vi "Pixels Per Micron For All FoV.vi"() -> ()   [LabVIEW 2020]
uses:
  <vilib>/vision/Measure.llb/Edge Options.ctl
  <vilib>/vision/Measure.llb/Edge Polarity.ctl
  <vilib>/Analysis/baseanly.llb/Mean (DBL).vi
  <vilib>/Utility/file.llb/Write Delimited Spreadsheet (DBL).vi
  <vilib>/vision/NI_Vision_Development_Module.lvlib
  <vilib>/Analysis/NI_AALBase.lvlib
panel:
  in  "Threshold Data":T1(array[cluster])=[{"Lower value"=140.0, "Upper value"=255.0, "Replace Value"=0.0, "Keep/Replace Value (Replace)"=FALSE}, {"Lower value"=140.0, "Upper value"=255.0, "Replace Value"=255.0, "Keep/Replace Value (Replace)"=TRUE}] {"Replace Value" format="%.2f"; "Upper value" format="%.2f"; "Lower value" format="%.2f"}
  out "output cluster":cluster{i32[], dbl[]}(graph)={[5, 6, 7, 8, 9, 10, 11, 12, 13, 14, 15, 16, 17, 18, 19, 20, 21, 22, 23, 24, 25, 26, 27, 28, 29, 30, 31, 32, 33, 34, 35, 36, 37, 38, 39, 40, 41, 42, 43, 44, 45, 46, 47, 48, 49, 50, 51, 52, 53, 54, 55, 56, 57, 58, 59, 60, 61, 62, 63, 64, 65, 66, 67, 68, 69, 70, 71, 72, 73, 74, 75, 76, 77, 78], [6.014901123046875, 0.0, 26.758624267578124, 14.584745788574219, 23.696197509765625, 0.0, 5.14136962890625, 33.5981689453125, 13.677774047851562, 24.873800659179686, 0.0, 30.73720703125, nan, 0.0, 35.932763671875, 0.0, nan, nan, 18.756075032552083, 0.0, 5.87806282043457, nan, 35.273126220703126, 2.967665100097656, 2.766326904296875, 9.08037872314453, nan, nan, nan, 38.17447204589844, nan, 0.0, 0.0, 12.061470031738281, nan, nan, nan, nan, nan, 0.0, nan, 23.260025024414062, nan, nan, nan, nan, 0.0, nan, 0.0, 0.0, 18.1035888671875, nan, nan, nan, 30.044448852539062, 8.698919677734375, nan, 0.0, nan, nan, nan, 47.926483154296875, nan, nan, nan, nan, nan, nan, nan, nan, nan, 17.186370849609375, nan, nan]}
  in  "Size & Tolerance":T2={"X Size"=5, "Y Size"=5, "% Tolerance"=10}
  in  "ROI":T3={"Global Rectangle"=[0, 0, 1023, 1023], "Contours"=[{"ID"=enum."External", "Type"=3, "Coordinates"=[0, 100, 1023, 900]}]} {"Contours"."Type" items=["No Selection", "Point", "Line", "Rectangle", "Oval", "Polygon", "Freehand Region", "Annulus", "Unused2", "Unused3", "Broken Line", "Freehand Line", "Rotated Rectangle"]}
  in  "Options":T6={"Search Direction"=0, "Edge Options"={"Edge Polarity"=1, "Kernel Size"=3, "Width"=7, "Minimum Edge Strength"=50.0, "Interpolation Type"=enum."Bilinear Fixed", "Data Processing Method"=enum."Average"}, "Show Search Area"=FALSE, "Show Search Lines"=FALSE, "Show Edges Found"=FALSE, "Show Result"=TRUE, "Search Area Color"=65280, "Search Lines Color"=255, "Edge Locations Color"=16776960, "Result Color"=16711680, "Overlay Group Name"=""} {"Search Direction" items=["Left to Right", "Right to Left", "Top to Bottom", "Bottom to Top"]; "Edge Options"."Edge Polarity" items=["All Edges", "Rising Edges", "Falling Edges"]; "Edge Options"."Minimum Edge Strength" format="%.2f"; "Edge Options"."Width" step=2; "Edge Options"."Kernel Size" step=2}
  out "Image":T7(plugin-control)
  in  "File Path":path=path "D:/Data/Calibration/2023/Zoom Cal 10um with correct Align/TIFFs"
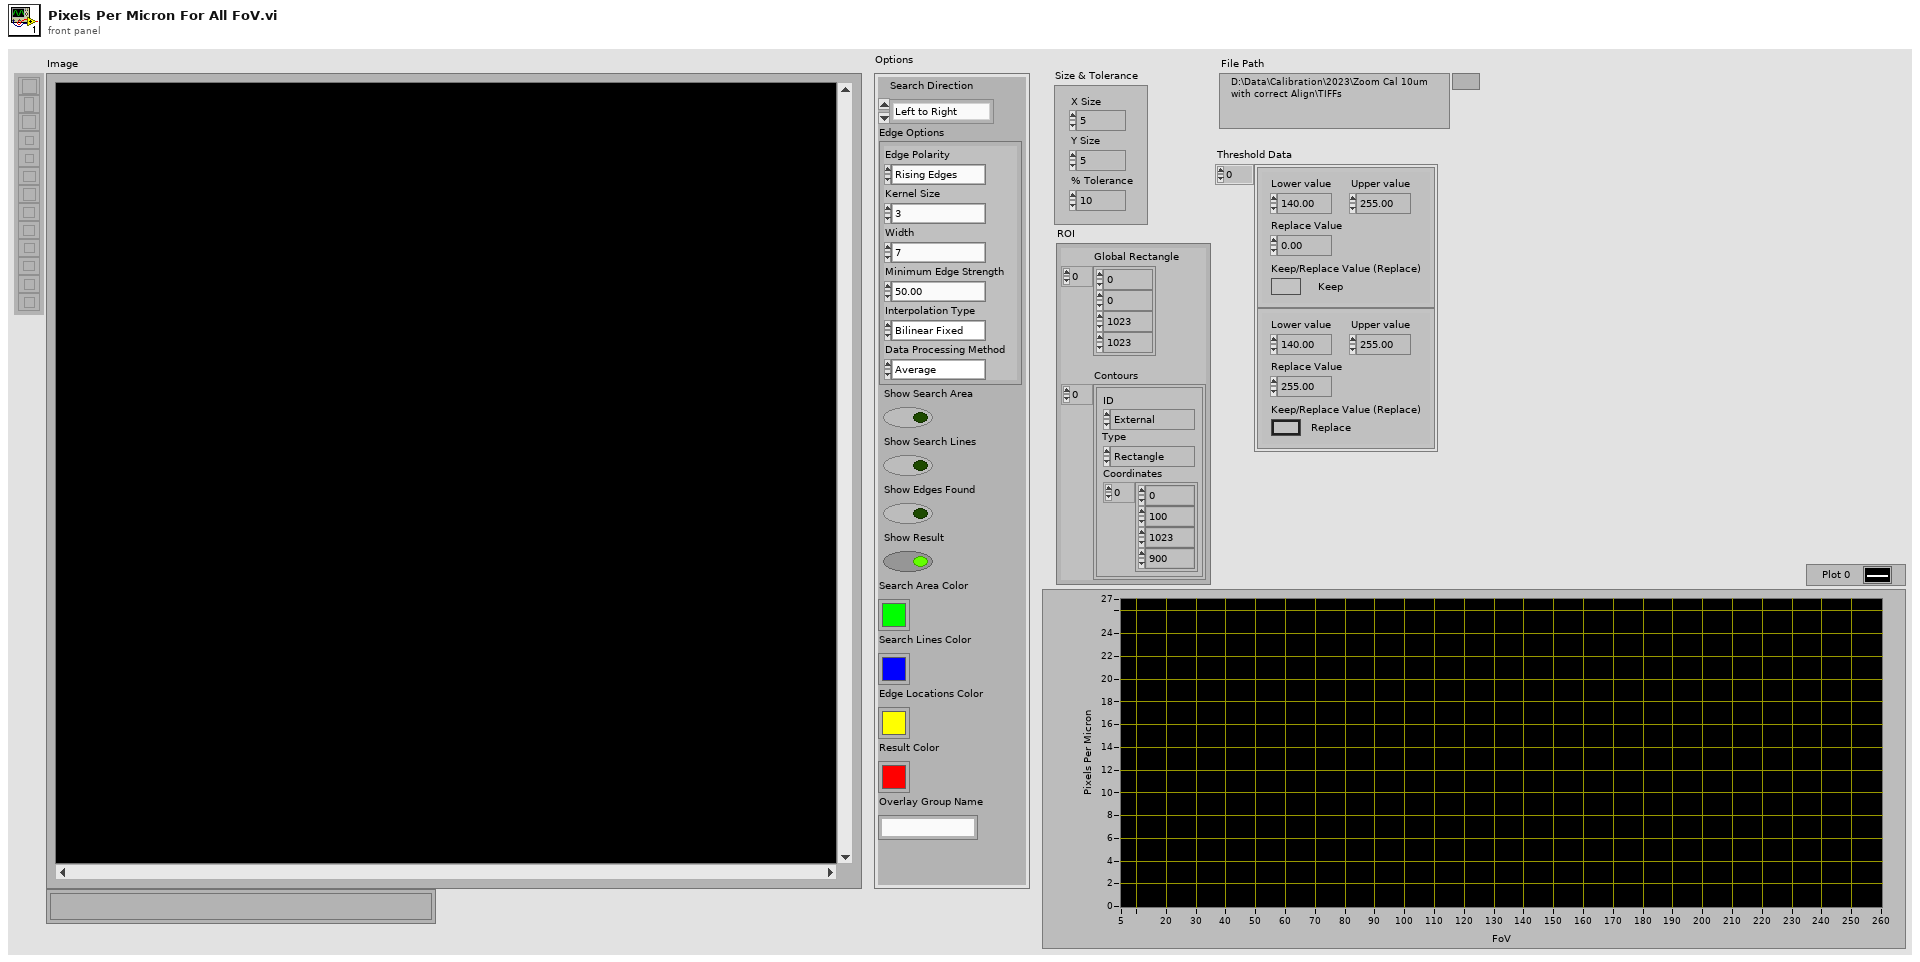
[diagram p1: front panel]
types:
  T1 = cluster{"Lower value":sgl, "Upper value":sgl, "Replace Value":sgl, "Keep/Replace Value (Replace)":bool}[]
  T2 = cluster{"X Size":i32, "Y Size":i32, "% Tolerance":i32}
  T3 = typedef "ROI Descriptor" = cluster{"Global Rectangle":i32[], "Contours":cluster{"ID":enum32{"External", "Internal"}, "Type":u32, "Coordinates":i32[]}[]}
  T4 = typedef "Edge Options.ctl" = cluster{"Edge Polarity":T5, "Kernel Size":u32, "Width":u32, "Minimum Edge Strength":sgl, "Interpolation Type":enum32{"Zero Order", "Bilinear", "Quadratic", "Cubic", "Bilinear Fixed"}, "Data Processing Method":enum32{"Average", "Median"}}
  T5 = typedef "Edge Polarity.ctl" = u32
  T6 = cluster{"Search Direction":u32, "Edge Options":T4, "Show Search Area":bool, "Show Search Lines":bool, "Show Edges Found":bool, "Show Result":bool, "Search Area Color":u32, "Search Lines Color":u32, "Edge Locations Color":u32, "Result Color":u32, "Overlay Group Name":string}
  T7 = typedef "IMAQ Image.ctl" = refnum<image>
  T8 = typedef "Image Type" = u32
  T9 = cluster{"ID":enum32{"External", "Internal"}, "Type":u32, "Coordinates":i32[]}[]
  T10 = cluster{"ID":enum32{"External", "Internal"}, "Type":u32, "Coordinates":i32[]}
  T11 = cluster{"Point1 (Pixels)":cluster{"X":sgl, "Y":sgl}, "Point2 (Pixels)":cluster{"X":sgl, "Y":sgl}, "Point1 (Real-World)":cluster{"X":sgl, "Y":sgl}, "Point2 (Real-World)":cluster{"X":sgl, "Y":sgl}, "Angle (Pixel)":dbl, "Angle (Real-World)":dbl, "Score":dbl, "Straightness":dbl, "Average SNR (db)":dbl, "Calibration Valid":bool}[]
  T12 = cluster{"Point1 (Pixels)":cluster{"X":sgl, "Y":sgl}, "Point2 (Pixels)":cluster{"X":sgl, "Y":sgl}, "Point1 (Real-World)":cluster{"X":sgl, "Y":sgl}, "Point2 (Real-World)":cluster{"X":sgl, "Y":sgl}, "Angle (Pixel)":dbl, "Angle (Real-World)":dbl, "Score":dbl, "Straightness":dbl, "Average SNR (db)":dbl, "Calibration Valid":bool}
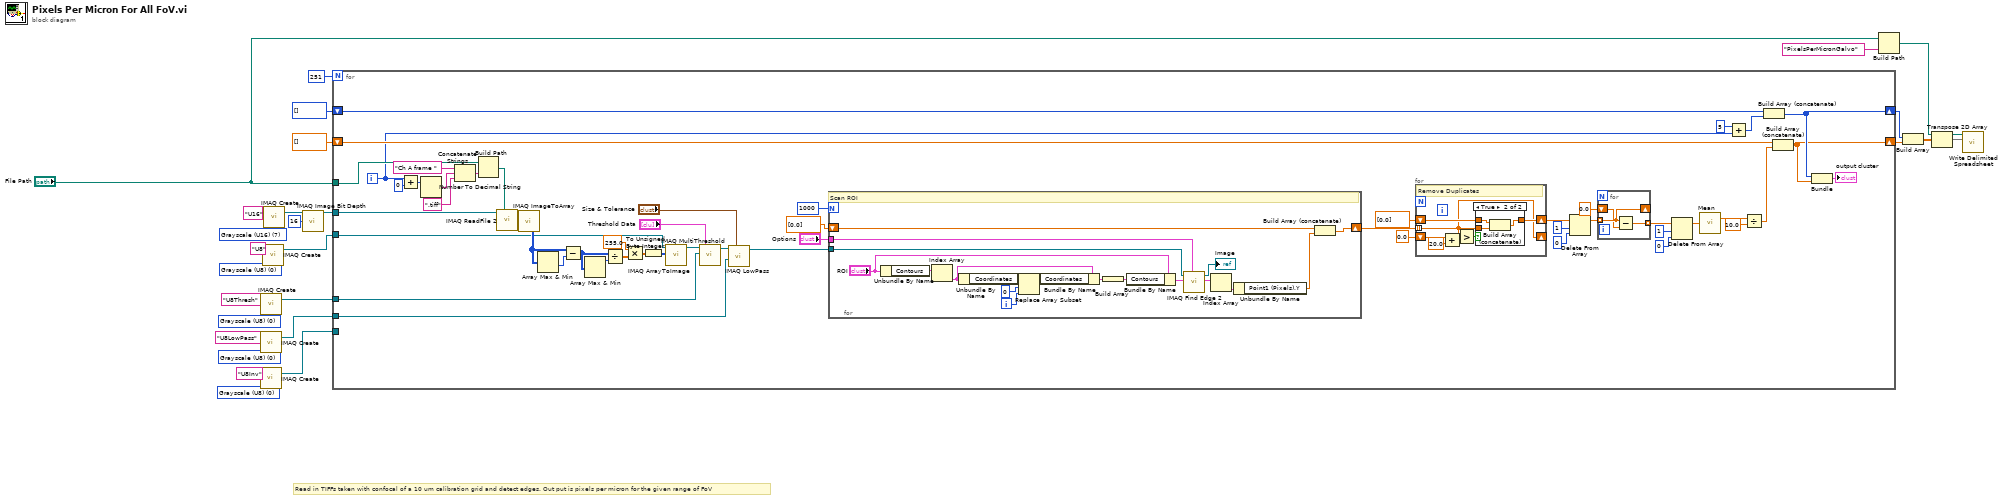
[diagram p0: block diagram]
diagram:
  w7 = T8 0 items=["Grayscale (U8)", "Grayscale (I16)", "Grayscale (SGL)", "Complex (CSG)", "RGB (U32)", "HSL (U32)", "RGB (U64)", "Grayscale (U16)"] ("Image Type")
  w15 = T8 0 items=["Grayscale (U8)", "Grayscale (I16)", "Grayscale (SGL)", "Complex (CSG)", "RGB (U32)", "HSL (U32)", "RGB (U64)", "Grayscale (U16)"] ("Image Type")
  w18 = T8 0 items=["Grayscale (U8)", "Grayscale (I16)", "Grayscale (SGL)", "Complex (CSG)", "RGB (U32)", "HSL (U32)", "RGB (U64)", "Grayscale (U16)"] ("Image Type")
  w21 = T8 0 items=["Grayscale (U8)", "Grayscale (I16)", "Grayscale (SGL)", "Complex (CSG)", "RGB (U32)", "HSL (U32)", "RGB (U64)", "Grayscale (U16)"] ("Image Type")
  w27 = T8 7 items=["Grayscale (U8)", "Grayscale (I16)", "Grayscale (SGL)", "Complex (CSG)", "RGB (U32)", "HSL (U32)", "RGB (U64)", "Grayscale (U16)"] ("Image Type")
  # "Read in TIFFs taken with confocal of a 10 um calibration grid and detect edges. Out put is pixels per micron for the given range of FoV"
  n1 = call "IMAQ Create"("Image Name"="U8LowPass", "Image Type"=w18) -> ("New Image"=w16:T7)  [unwired: 3 in, 1 out]
  n2 = call "IMAQ Create"("Image Name"="U8Inv", "Image Type"=w15) -> ("New Image"=w13:T7)  [unwired: 3 in, 1 out]
  n3 = call "IMAQ Create"("Image Name"="U8Thresh", "Image Type"=w7) -> ("New Image"=w5:T7)  [unwired: 3 in, 1 out]
  n4 = call "IMAQ Create"("Image Name"="U8", "Image Type"=w21) -> ("New Image"=w19:T7)  [unwired: 3 in, 1 out]
  n5 = call "IMAQ Create"("Image Name"="U16", "Image Type"=w27) -> ("New Image"=w24:T7)  [unwired: 3 in, 1 out]
  n6 = call "IMAQ Image Bit Depth"("Image"=w24, "Bit Depth (0)"=u32 16) -> ("Image Out"=w23:T7)  [unwired: 11 in, 2 out]
  n7 = for {
    N: 251 -> [_]
    tunnel: "File Path" -> [w79]
    tunnel: w23 -> [w69]
    tunnel: w19 -> [w61]
    tunnel: w16 -> [w43]
    tunnel: w13 -> [_]
    shift-right: [w36] -> w2
    shift-left: dbl[] [] -> [w56]
    shift-right: [w37] -> w1
    shift-left: i32[] [] -> [w38]
    tunnel: w5 -> [w33]
    i -> [w41]
    n8 = Add(x=w41, y=0) -> (x+y=w71:i32)
    n9 = Number To Decimal String(number=w71) -> (decimal integer string=w75:string)  [unwired: 1 in]
    n10 = Concatenate Strings("Ch A frame ", w75, ".tiff") -> (w76:string)
    n11 = Build Path(base path=w79, name or relative path=w76) -> (appended path=w78:path)
    n12 = call "IMAQ ReadFile 2"("File Path"=w78, "Image"=w69) -> ("Image Out"=w68:T7)  [unwired: 5 in, 4 out]
    n13 = call "IMAQ ImageToArray"("Image"=w68) -> ("Image Pixels (U16)"=w67:u16[][])  [unwired: 3 in, 4 out]
    n14 = Array Max & Min(array=w67) -> (min value=w66:u16)  [unwired: 3 out]
    n15 = Subtract(x=w67, y=w66) -> (x-y=w65:u16[][])
    n16 = Array Max & Min(array=w65) -> (max value=w64:u16)  [unwired: 3 out]
    n17 = Divide(x=w65, y=w64) -> (x/y=w63:dbl[][])
    n18 = Multiply(x=255.0, y=w63) -> (x*y=w60:dbl[][])
    n19 = To Unsigned Byte Integer(number=w60) -> (unsigned 8bit integer=w62:u8[][])
    n20 = call "IMAQ ArrayToImage"("Image Pixels (U8)"=w62, "Image"=w61) -> ("Image Out"=w31:T7)  [unwired: 8 in, 1 out]
    n21 = call "IMAQ MultiThreshold"("Threshold Data"="Threshold Data", "Image Dst"=w33, "Image Src"=w31) -> ("Image Dst Out"=w30:T7)  [unwired: 2 in, 1 out]
    n22 = call "IMAQ LowPass"("Image Src"=w30, "Size & Tolerance"="Size & Tolerance", "Image Dst"=w43) -> ("Image Dst Out"=w29:T7)  [unwired: 4 in, 1 out]
    n23 = for {
      N: 1000 -> [_]
      tunnel: "Options" -> [w111]
      tunnel: w29 -> [w98]
      shift-right: [w96] -> w47
      shift-left: sgl[] [0.0] -> [w95]
      i -> [w108]
      # "Scan ROI"
      n24 = Unbundle By Name("ROI") -> ("Contours"=w107:T9)
      n25 = Index Array(array=w107) -> (element=w104:T10)  [unwired: 1 in]
      n26 = Unbundle By Name(w104) -> ("Coordinates"=w106:i32[])
      n27 = Replace Array Subset(array=w106, new element=w108, index=0) -> (w105:i32[])
      n28 = Bundle By Name(cluster=w104, "Coordinates"=w105) -> (w103:T10)
      n29 = Build Array(w103) -> (w102:T9)
      n30 = Bundle By Name(cluster="ROI", "Contours"=w102) -> (w100:T3)
      n31 = call "IMAQ Find Edge 2"("Options"=w111, "ROI Descriptor"=w100, "Image"=w98) -> ("Straight Edges"=w99:T11, "Image Out"=→"Image":T7)  [unwired: 5 in, 2 out]
      n32 = Index Array(array=w99) -> (element=w97:T12)  [unwired: 1 in]
      n33 = Unbundle By Name(w97) -> ("Point1 (Pixels).Y"=w94:sgl)
      n34 = Build Array (concatenate)(w95, w94) -> (w96:sgl[])
    }
    n35 = for {
      tunnel: w47 -> [w81] mode=indexing
      shift-right: [w81] -> _
      shift-left: sgl 0.0 ("X") -> [w83]
      shift-right: [w84] -> w46
      shift-left: sgl[] [0.0] -> [w85]
      # "Remove Duplicates"
      n36 = Add(x=w83, y=sgl 20.0) -> (x+y=w80:sgl)
      n37 = Greater?(x=w81, y=w80) -> (0:w86:bool)
      n38 = case shown="True" w86 {
        tunnel: w81 -> [_ w90]
        tunnel: w85 -> [w87 w89]
        tunnel: [w87 w88] -> w84
        frame False {
        }
        frame True {
          n39 = Build Array (concatenate)(w89, w90) -> (w88:sgl[])
        }
      }
    }
    n40 = Delete From Array(array=w46, length=1, index=0) -> (array with subset deleted=w52:sgl[])  [unwired: 1 out]
    n41 = for {
      shift-right: [w92] -> _
      shift-left: sgl 0.0 ("X") -> [w91]
      tunnel: w52 -> [w92] mode=indexing
      tunnel: [w93] -> w49 mode=indexing
      n42 = Subtract(x=w92, y=w91) -> (x-y=w93:sgl)
    }
    n43 = Delete From Array(array=w49, length=1, index=0) -> (array with subset deleted=w48:sgl[])  [unwired: 1 out]
    n44 = call-poly <vilib>:"Mean.vi"("X"=w48) -> ("mean"=w55:dbl)  [unwired: 1 out]
    n45 = Add(x=5, y=w41) -> (x+y=w39:i32)
    n46 = Divide(x=w55, y=10.0) -> (x/y=w35:dbl)
    n47 = Build Array (concatenate)(w38, w39) -> (w37:i32[])
    n48 = Build Array (concatenate)(w56, w35) -> (w36:dbl[])
    n49 = Bundle(w37, w36) -> (→"output cluster":cluster{i32[], dbl[]})  [unwired: 1 in]
  }
  n50 = Build Path(base path="File Path", name or relative path="PixelsPerMicronGalvo") -> (appended path=w11:path)
  n51 = Build Array(w1, w2) -> (w9:dbl[][])
  n52 = Transpose 2D Array(2D array=w9) -> (transposed array=w8:dbl[][])
  n53 = call-poly <vilib>:"Write Delimited Spreadsheet.vi"("file path (dialog if empty)"=w11, "2D data"=w8) -> ()  [unwired: 12 in, 2 out]
